vi "Popup - Break Out Menu.vi"(8 "error in (no error)":errorcluster) -> (0 "error out":errorcluster, 1 "Edit SubTests?":bool, 2 "Main Menu?":bool, 4 "Exit?":bool)   [LabVIEW 2018]
doc: "This is the dialog used by the user to select an APU to test."
panel:
  in  "Exit":bool
  in  "Main Menu":bool
  # "What would you like to do?"
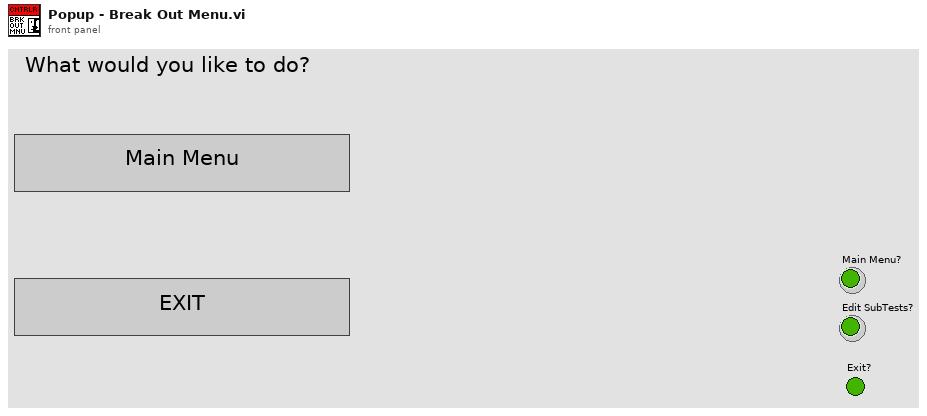
[diagram p1: front panel]
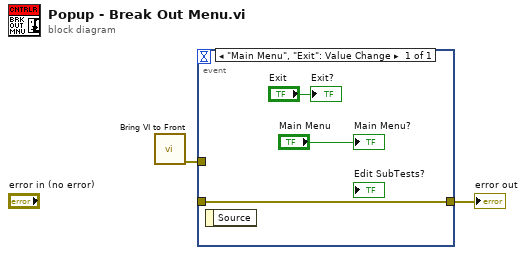
[diagram p0: block diagram]
diagram:
  n1 = call "Bring VI to Front.vi"() -> ("error out"=w4:errorcluster)  [unwired: 11 in]
  n2 = event shown="[0] \"Main Menu\", \"Exit\": Value Change" {
    selector: _ -> [_]
    dyn-events: _ -> [_]
    timeout: _ -> [_]
    tunnel: w4 -> [_]
    tunnel: [w5] -> w2
    tunnel: [w5] -> w1
    event "Main Menu", "Exit": Value Change {
      n3 = event-data() -> ()  [unwired: 1 in, 1 out]
      "Main Menu?" <- "Main Menu"
      "Exit?" <- "Exit"
    }
  }
  "error out" <- w1
